vi "Get SMO Vendor.vi"(8 "error in (no error)":errorcluster, 11 "instrument.PPMS in":refnum<class "instrument.PPMS.lvclass">) -> (0 "error out":errorcluster, 2 "SMO Vendor":string, 3 "instrument.PPMS out":refnum<class "instrument.PPMS.lvclass">)   [LabVIEW 2019, in "instrument.PPMS.lvclass"]
doc: "Override this VI to return the vendor or manufacturer of your Instrument"
uses:
  instrument.PPMS.lvclass
  <userlib>/LevyLab/Instrument Framework/Instrument Types/Cryostat/Instrument.Cryostat.lvclass
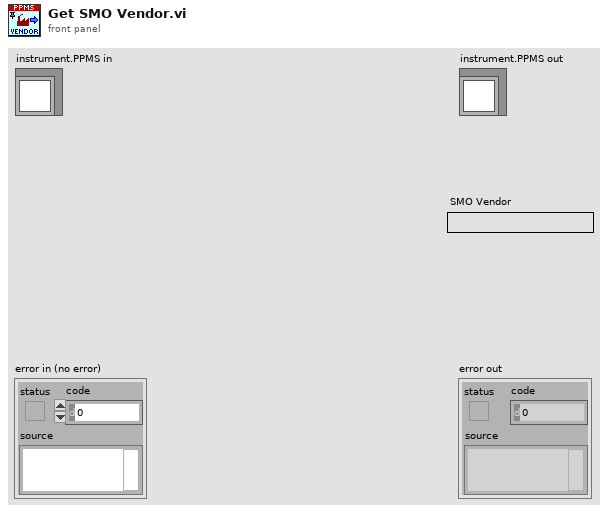
[diagram p1: front panel]
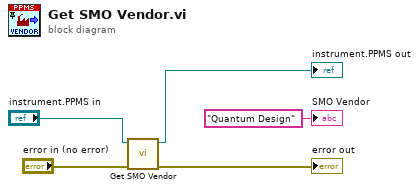
[diagram p0: block diagram]
diagram:
  n1 = call-parent "Get SMO Vendor.vi"("error in (no error)"="error in (no error)", "Instrument in"="instrument.PPMS in") -> ("error out"=→"error out":errorcluster, "Instrument out"=→"instrument.PPMS out":refnum<class "instrument.PPMS.lvclass">)  [unwired: 7 in, 1 out]
  "SMO Vendor" <- "Quantum Design" ("SMO Vendor")
